vi "Drop Continuous Query.vi"(0 "InfluxDB in":refnum<class "Client.lvclass">, 5 "Database name":string, 11 "error in (no error)":errorcluster) -> (4 "InfluxDB out":refnum<class "Client.lvclass">, 15 "error out":errorcluster)   [LabVIEW 2018, in "InfluxDB Client.lvlib" / "Client.lvclass"]
doc: "Creates a database."
uses:
  Client.lvclass
panel:
  in  "Continuos query name":string
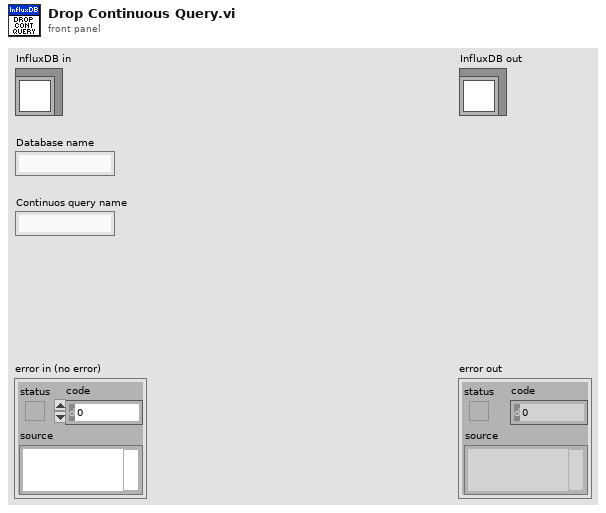
[diagram p1: front panel]
types:
  T1 = typedef "Dictionary Object RefNum__ogtk.ctl" = refnum<k1>
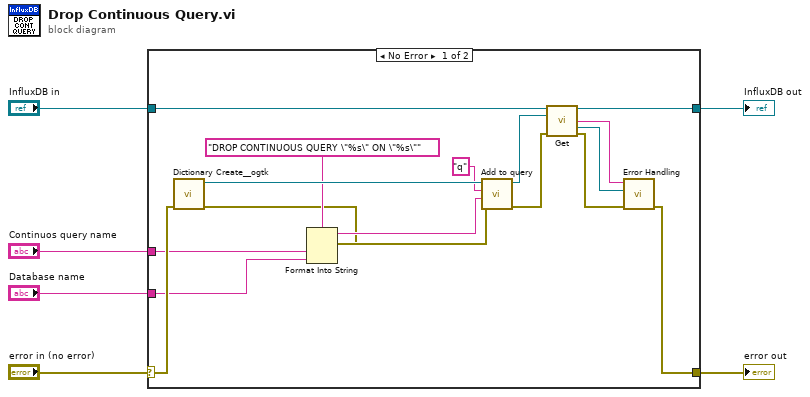
[diagram p0: block diagram]
diagram:
  n1 = case shown="No Error" "error in (no error)" {
    selector: "error in (no error)" -> [w14 w25]
    tunnel: [w9 w25] -> w5
    tunnel: [w22 w24] -> w3
    tunnel: "InfluxDB in" -> [w23 w24]
    tunnel: "Database name" -> [w7 _]
    tunnel: "Continuos query name" -> [w8 _]
    frame No Error {
      n2 = call <userlib>:"Dictionary Create__ogtk.vi"("error in (no error)"=w14) -> ("error out"=w13:errorcluster, "dictionary out"=w21:T1)  [unwired: 9 in]
      n3 = Format Into String(format string="DROP CONTINUOUS QUERY \"%s\" ON \"%s\"" ("Username"), error in=w13, w8, w7) -> (resulting string=w17:string, error out=w16:errorcluster)  [unwired: 1 in]
      n4 = call "Add to query.vi"("error in (no error)"=w16, "Value"=w17, "Parameter"="q" ("String"), "Query in"=w21) -> ("error out"=w15:errorcluster, "Query out"=w19:T1)  [unwired: 6 in]
      n5 = call "Get.vi"("InfluxDB Client in"=w23, "Query"=w19, "error in (no error)"=w15) -> ("InfluxDB Client out"=w22:refnum<class "Client.lvclass">, "Status code"=w12:string, "Headers"=w11:T1, "error out"=w10:errorcluster)  [unwired: 8 in, 1 out]
      n6 = call "Error Handling.vi"("error in (no error)"=w10, "HTTP headers"=w11, "HTTP status code"=w12) -> ("error out"=w9:errorcluster)  [unwired: 8 in]
    }
    frame Error {
    }
  }
  "error out" <- w5
  "InfluxDB out" <- w3
